vi "ECS-100X - Next Cycle Control.vi"(10 "CAS FPGA Ref":T1) -> ()   [LabVIEW 2015, in "ECS-RT.lvlib"]
uses:
  ECS-RT.lvlib
  <vilib>/addons/Combustion Analysis System/FPGA/CAS - FGPA - Reference.ctl
  Typedefs/MISC/50% MFB - Results.ctl
  <vilib>/addons/Combustion Analysis System/Real-Time/Globals/CAS - Control.vi
  Globals/RT Data.vi
  <vilib>/addons/Combustion Analysis System/Real-Time/Globals/Results/CAS - Results - All Results.vi
  <vilib>/addons/Combustion Analysis System/Real-Time/Globals/CAS - Queues.vi
  <vilib>/addons/Combustion Analysis System/Real-Time/Globals/Setup/CAS - Setup - Engine Geometry.vi
  Globals/Next Cycle Globals.vi
  <vilib>/Utility/error.llb/Error Cluster From Error Code.vi
  <vilib>/rvi/errors/niLvFpgaAdjustHostInterfaceError.vi
  <vilib>/rvi/interface/nirviReadWriteControl/nirviReadWriteControl.xnode
  ECS-Shared.lvlib
  NiFpgaLv.dll
  <vilib>/rvi/interface/Simulation/niFpgaSimulationCallBeginRW.vi
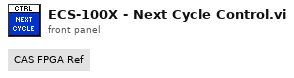
[diagram p1: front panel]
types:
  T1 = typedef "CAS - FGPA - Reference.ctl" = refnum<k20>
  T2 = typedef "ECS-Shared.lvlib/RT Data.ctl" = cluster{"Refs":T3, "EPT":T5, "Raw Inputs":T7, "Control Inputs":T14, "Control Outputs":T17, "Raw Outputs":T20}
  T3 = typedef "ECS-Shared.lvlib/FPGA Refs.ctl" = cluster{"FPGA 1":T4, "FPGA 2":T4}
  T4 = typedef "ECS-Shared.lvlib/Generic FPGA Ref.ctl" = refnum<k20>
  T5 = typedef "ECS-Shared.lvlib/EPT Cluster.ctl" = cluster{"MaxCAD":sgl, "EPT Sim Enabled":bool, "EPTxData":T6}
  T6 = typedef "EPTx - RevA - RT.lvlib/EPTxData.ctl" = cluster{"Sync":bool, "CurrentCAD":sgl, "Speed [RPM]":sgl, "Config":bool, "Rcvg Primary":bool, "Stall":bool, "Overflow":bool, "Ratio Error":bool, "Pattern Error":bool, "Aux Warning":bool, "Watchdog Error":bool}
  T7 = typedef "ECS-Shared.lvlib/Raw Inputs.ctl" = cluster{"NI9752s":T8[], "NI9757s":T10[], "NI9411s":T11[], "NI9220s":T12[], "VRHalls":T13[]}
  T8 = typedef "ECS-Shared.lvlib/NI9752.ctl" = cluster{"Voltage [V]":sgl[], "Resistance [Ohm]":sgl[], "PPWData VR1":T9, "PPWData VR2":T9, "PPWData Hall1":T9, "PPWData Hall2":T9}
  T9 = typedef "ECS-Shared.lvlib/PPWData.ctl" = cluster{"Period":u32, "PulseWidth":u32, "Stopped":bool}
  T10 = typedef "ECS-Shared.lvlib/NI9757.ctl" = cluster{"UEGO1":cluster{"Lambda":sgl, "Phi":sgl, "AF_Ratio":sgl, "Ip":sgl, "Temp":sgl, "Hot":bool}, "UEGO2":cluster{"Lambda":sgl, "Phi":sgl, "AF_Ratio":sgl, "Ip":sgl, "Temp":sgl, "Hot":bool}, "EGO1":cluster{"Status":enum16{"COLD SENSOR", "FOULED SENSOR", "RICH", "LEAN"}, "SensorV":sgl}, "EGO2":cluster{"Status":enum16{"COLD SENSOR", "FOULED SENSOR", "RICH", "LEAN"}, "SensorV":sgl}, "EGO3":cluster{"Status":enum16{"COLD SENSOR", "FOULED SENSOR", "RICH", "LEAN"}, "SensorV":sgl}, "EGO4":cluster{"Status":enum16{"COLD SENSOR", "FOULED SENSOR", "RICH", "LEAN"}, "SensorV":sgl}}
  T11 = typedef "ECS-Shared.lvlib/NI9411.ctl" = cluster{"PPWData 0":T9, "PPWData 1":T9, "PPWData 2":T9, "PPWData 3":T9, "PPWData 4":T9, "PPWData 5":T9}
  T12 = typedef "ECS-Shared.lvlib/NI9220.ctl" = cluster{"AI 0":sgl, "AI 1":sgl, "AI 2":sgl, "AI 3":sgl, "AI 4":sgl, "AI 5":sgl, "AI 6":sgl, "AI 7":sgl, "AI 8":sgl, "AI 9":sgl, "AI 10":sgl, "AI 11":sgl, "AI 12":sgl, "AI 13":sgl, "AI 14":sgl, "AI 15":sgl}
  T13 = typedef "ECS-Shared.lvlib/VRHall.ctl" = cluster{"PPWData 0":T9, "PPWData 1":T9, "PPWData 2":T9, "PPWData 3":T9, "PPWData 4":T9, "PPWData 5":T9}
  T14 = typedef "ECS-Shared.lvlib/Control Inputs.ctl" = cluster{"Engine Speed [RPM]":sgl, "Engine Status":T15, "Load Control \nMode":T16, "dt(s)":sgl, "Number of Cylinders":u8, "Engine Displacement [cc]":sgl, "StoichAFR":sgl, "Q.LHV Fuel [kJ/kg]":sgl, "BattV PSU [V]":sgl, "12V PSU [V]":sgl, "5V PSU [V]":sgl, "Pedal Position [%]":sgl, "Oil Pressure [kPa]":sgl, "Oil Temp [C]":sgl, "Oil Level [%]":sgl, "Engine Coolant Temp (ECT) [C]":sgl, "Engine Coolant Pressure [kPa]":sgl, "Rail Pressure [bar]":sgl, "Fuel Pressure [kPa]":sgl, "Fuel Temp [C]":sgl, "Vacuum Pressure [kPa]":sgl, "Throttle Position [%]":sgl, "Cam1 Advance [CAD]":sgl, "Cam2 Advance [CAD]":sgl, "Cam3 Advance [CAD]":sgl, "Cam4 Advance [CAD]":sgl, "CA50 Control Output [CAD]":sgl[], "CA50 Control Output Valid":bool[], "Intake Air Temp (IAT) [C]":sgl, "Barometric Air Pressure [kPa]":sgl, "Intake Air Rel. Humidity [%]":sgl, "Mass Air Flow (MAF) [kg/hr]":sgl, "Turbo Inlet Air Pressure [kPa]":sgl, "Turbo Inlet Air Temp [C]":sgl, "Turbo Outlet Air Pressure [kPa]":sgl, "Turbo Outlet Air Temp [C]":sgl, "CAC Outlet Pressure [kPa]":sgl, "CAC Outlet Temp [C]":sgl, "Intake Manifold Pressure (MAP) [kPa]":sgl, "Intake Manifold Temp (MAT) [C]":sgl, "Exhaust Manifold Pressure [kPa]":sgl, "Exhaust Manifold Temp [C]":sgl, "HighP EGR Cooler Outlet Pressure [kPa]":sgl, "HighP EGR Cooler Outlet Temp [C]":sgl, "HighP EGR Differential Pressure [kPa]":sgl, "HighP EGR Valve Position [%]":sgl, "Turbo Outlet Exhaust Pressure [kPa]":sgl, "Turbo Outlet Exhaust Temp [C]":sgl, "VGT Position 1 [%]":sgl, "VGT Position 2 [%]":sgl, "Turbo Speed 1 [RPM]":sgl, "Turbo Speed 2 [RPM]":sgl, "LowP EGR Differential Pressure [kPa]":sgl, "LowP EGR Valve Position [%]":sgl, "UEGO1Lambda":sgl, "UEGO1_Hot":bool, "UEGO2Lambda":sgl, "UEGO2_Hot":bool, "Knock Intensity":sgl[], "Knock":bool[]}
  T15 = typedef "ECS-Shared.lvlib/Engine Status.ctl" = enum16{"OFF", "STALLED", "CRANKING", "RUNNING", "ACCEL", "DECEL", "SAFE"}
  T16 = typedef "ECS-Shared.lvlib/Load Control Mode.ctl" = enum16{"No Governor", "Min Speed Governor", "Max Speed Governor"}
  T17 = typedef "ECS-Shared.lvlib/Control Outputs.ctl" = cluster{"Pedal Desired [%]":sgl, "MEP Desired [bar]":sgl, "Fuel Desired [mg/cyc]":sgl, "Intake MAP Desired [kPa]":sgl, "Cam1 Advance Setpoint [CAD]":sgl, "Cam2 Advance Setpoint [CAD]":sgl, "HighP EGR Position Setpoint [%Open]":sgl, "LowP EGR Position Setpoint [%Open]":sgl, "Rail Pressure Setpoint [bar]":sgl, "Wastegate1 Position Setpoint [%Open]":sgl, "Wastegate2 Position Setpoint [%Open]":sgl, "VGT1 Position Setpoint [%Open]":sgl, "VGT2 Position Setpoint [%Open]":sgl, "Throttle1 Position Setpoint [%Open]":sgl, "Throttle2 Position Setpoint [%Open]":sgl, "TurboBPV Position Setpoint [%Open]":sgl, "Spark Dwells [msec]":sgl[], "Spark Timings [DBTDC]":sgl[], "PFI Quantities [mg/inj]":sgl[], "PFI Timings [DBTDC]":sgl[], "DI Quantities [mg/inj]":T18[], "DI Timings [DBTDC]":T19[]}
  T18 = typedef "ECS-Shared.lvlib/Injection Quantity.ctl" = cluster{"Pilot1Quantity [mg/inj]":sgl, "Pilot2Quantity [mg/inj]":sgl, "MainQuantity [mg/inj]":sgl, "Post1Quantity [mg/inj]":sgl, "Post2Quantity [mg/inj]":sgl}
  T19 = typedef "ECS-Shared.lvlib/Injection Timing.ctl" = cluster{"Pilot1SOI [DBTDC]":sgl, "Pilot2SOI [DBTDC]":sgl, "MainSOI [DBTDC]":sgl, "Post1SOI [DBTDC]":sgl, "Post2SOI [DBTDC]":sgl}
  T20 = typedef "ECS-Shared.lvlib/Raw Outputs.ctl" = cluster{"9751-1":T21, "9751-2":T21, "9751-3":T21, "9751-4":T21, "9754-1":T23, "9754-2":T23, "9758-1":T25, "9758-2":T25, "9759-1":T28}
  T21 = typedef "ECS-Shared.lvlib/NI9751.ctl" = cluster{"DI1":T22, "DI2":T22, "DI3":T22}
  T22 = typedef "ECS-Shared.lvlib/DI.ctl" = cluster{"Window_Start (DBTDC)":sgl, "Window_End (DBTDC)":sgl, "Enable_Inj1":bool, "Duration_Inj1 (msec)":sgl, "Timing_Inj1 (DBTDC)":sgl, "Enable_Inj2":bool, "Duration_Inj2 (msec)":sgl, "Timing_Inj2 (DBTDC)":sgl, "Enable_Inj3":bool, "Duration_Inj3 (msec)":sgl, "Timing_Inj3 (DBTDC)":sgl, "Enable_Inj4":bool, "Duration_Inj4 (msec)":sgl, "Timing_Inj4 (DBTDC)":sgl, "Enable_Inj5":bool, "Duration_Inj5 (msec)":sgl, "Timing_Inj5 (DBTDC)":sgl}
  T23 = typedef "ECS-Shared.lvlib/NI9754.ctl" = cluster{"ESTTL 1":T24, "ESTTL 2":T24, "ESTTL 3":T24, "ESTTL 4":T24, "ESTTL 5":T24, "ESTTL 6":T24, "ESTTL 7":T24, "ESTTL 8":T24}
  T24 = typedef "ECS-Shared.lvlib/ESTTL.ctl" = cluster{"Timing (DBTDC)":sgl, "Dwell (ms)":sgl}
  T25 = typedef "ECS-Shared.lvlib/NI9758.ctl" = cluster{"LS 1":T26, "LS 2":T26, "LS 3":T26, "LS 4":T26, "PFI 1":T27, "PFI 2":T27, "PFI 3":T27, "PFI 4":T27}
  T26 = typedef "ECS-Shared.lvlib/LS.ctl" = cluster{"Enable":bool, "Freq [Hz]":sgl, "DutyCyc [%]":sgl}
  T27 = typedef "ECS-Shared.lvlib/PFI.ctl" = cluster{"Position Mode":bool, "Timing (DBTDC)":sgl, "Pulse Width (ms)":sgl}
  T28 = typedef "ECS-Shared.lvlib/NI9759.ctl" = cluster{"THR1-1 DC [%]":sgl, "THR1-1 Setpoint [% Open]":sgl, "THR1-2 DC [%]":sgl, "THR1-2 Setpoint [% Open]":sgl}
  T29 = cluster{"Start Time [ns]":u64, "FPGA Time [ns]":u64, "Cycle":u32, "Cycle Period [Ticks]":u32}
  T30 = typedef "ECS-Shared.lvlib/50% MFB - Results.ctl" = cluster{"Result Valid":bool, "Time [ns]":u64, "50% Mass Fraction [CAD]":sgl, "Current Angle [DBTDC]":sgl}
  T31 = typedef "CAS - Results - All Results.ctl" = cluster{"Cycle Results":T32, "Pegging Results":T33, "Basic Results":T34, "Mean Effective Pressure Results":T35, "Injection Results":T36, "Spark Results":T37, "Heat Release Results":T38, "Combustion Noise Results":T39, "Misfire Results":T40, "Cam Results":T41, "Synchronous Pump Results":T42, "PWM Results":T43[], "Knock Results":T44, "FPGA Results":T45[], "Medium Speed Results":T46[], "User Results":T47[], "Slow Speed Results":T48[]}
  T32 = typedef "CAS - Results - Cycle.ctl" = cluster{"Enabled":bool, "Error Code":i32, "Cylinder":i32, "Speed [RPM]":sgl, "Time [ns]":u64, "Cycle":u32}
  T33 = typedef "CAS - Results - Pegging.ctl" = cluster{"Enabled":bool, "Error Code":i32, "Pegging Value [kPa]":sgl}
  T34 = typedef "CAS - Results - Basic.ctl" = cluster{"Enabled":bool, "Error Code":i32, "Peak Pressure [kPa abs]":sgl[], "Peak Pressure Location [CAD]":sgl[], "Max Pressure Rise Rate [kPa/CAD]":sgl[], "Max Pressure Rise Rate Location [CAD]":sgl[], "Polytropic Compression":sgl[], "Polytropic Expansion":sgl[], "Intake Pressure [kPa abs]":sgl, "Exhaust Pressure [kPa abs]":sgl, "TDC Probe Location [CAD]":sgl}
  T35 = typedef "CAS - Results - Mean Effective Pressure.ctl" = cluster{"Enabled":bool, "Error Code":i32, "Gross Mean Effective Pressure [kPa]":sgl[], "Pumping Mean Effective Pressure [kPa]":sgl, "Net Mean Effective Pressure [kPa]":sgl, "Indicated Power [kW]":sgl}
  T36 = typedef "CAS - Results - Injection.ctl" = cluster{"Enabled":bool, "Error Code":i32, "Number of Injections":u8, "Start of Injection [CAD]":sgl[], "Injection Duration [ms]":sgl[], "Injection Fuel Flow [mg/Inj]":sgl[], "Cycle Fuel Flow [mg/Cycle]":sgl}
  T37 = typedef "CAS - Results - Spark.ctl" = cluster{"Enabled":bool, "Error Code":i32, "Number of Sparks":u8, "Spark [CAD]":sgl[], "Dwell [ms]":sgl[], "Restrikes":sgl[], "Restrike Delay [ms]":sgl[], "Restrike Dwell [ms]":sgl[]}
  T38 = typedef "CAS - Results - Heat Release.ctl" = cluster{"Enabled":bool, "Error Code":i32, "5% Mass Fraction Burned [CAD]":sgl[], "10% Mass Fraction Burned [CAD]":sgl[], "50% Mass Fraction Burned [CAD]":sgl[], "75% Mass Fraction Burned [CAD]":sgl[], "90% Mass Fraction Burned [CAD]":sgl[], "Max Heat Release Rate [J/CAD]":sgl[], "Max Heat Release Rate Location [CAD]":sgl[]}
  T39 = typedef "CAS - Results - Combustion Noise.ctl" = cluster{"Enabled":bool, "Error Code":i32, "Noise [db]":sgl}
  T40 = typedef "CAS - Results - Misfire.ctl" = cluster{"Enabled":bool, "Error Code":i32, "Misfire":sgl}
  T41 = typedef "CAS - Results - Cam.ctl" = cluster{"Enabled":bool, "Error Code":i32, "Intake Cam Phase [CAD]":sgl, "Intake Phase [CAD]":sgl[], "Exhaust Cam Phase [CAD]":sgl, "Exhaust Phase [CAD]":sgl[]}
  T42 = typedef "CAS - Results - Synchronous Pump.ctl" = cluster{"Enabled":bool, "Error Code":i32, "Number of Pumps":u8, "Pump Start [CAD]":sgl[], "Pump End [CAD]":sgl[], "Pump Duration [CAD]":sgl[]}
  T43 = typedef "CAS - Results - PWM.ctl" = cluster{"Name":string, "Value":sgl}
  T44 = typedef "CAS - Results - Knock.ctl" = cluster{"Enabled":bool, "Error Code":i32, "Knock":sgl, "Peak-To-Peak":sgl}
  T45 = typedef "CAS - Results - FPGA.ctl" = cluster{"Name":string, "Value":sgl}
  T46 = typedef "CAS - Results - Medium Speed.ctl" = cluster{"Name":string, "Value":sgl}
  T47 = typedef "CAS - Results - User.ctl" = cluster{"Name":string, "Value":sgl}
  T48 = typedef "CAS - Results - Slow Speed.ctl" = cluster{"Name":string, "Value":sgl}
  T49 = typedef "DCAT.lvlib/DCAT - Results - All Results.ctl" = cluster{"Cycle Results":T50, "Pegging Results":T51, "Basic Results":T52, "Mean Effective Pressure Results":T53, "Injection Results":T54, "Spark Results":T55, "Heat Release Results":T56, "Combustion Noise Results":T57, "Misfire Results":T58, "Cam Results":T59, "Synchronous Pump Results":T60, "PWM Results":T61[], "Knock Results":T62, "FPGA Results":T63[], "Medium Speed Results":T64[], "User Results":T65[], "Slow Speed Results":T66[]}
  T50 = typedef "DCAT.lvlib/DCAT - Results - Cycle.ctl" = cluster{"Enabled":bool, "Error Code":i32, "Cylinder":i32, "Speed [RPM]":sgl, "Time [ns]":u64, "Cycle":u32}
  T51 = typedef "DCAT.lvlib/DCAT - Results - Pegging.ctl" = cluster{"Enabled":bool, "Error Code":i32, "Pegging Value [kPa]":sgl}
  T52 = typedef "DCAT.lvlib/DCAT - Results - Basic.ctl" = cluster{"Enabled":bool, "Error Code":i32, "Peak Pressure [kPa abs]":sgl[], "Peak Pressure Location [CAD]":sgl[], "Max Pressure Rise Rate [kPa/CAD]":sgl[], "Max Pressure Rise Rate Location [CAD]":sgl[], "Polytropic Compression":sgl[], "Polytropic Expansion":sgl[], "Intake Pressure [kPa abs]":sgl, "Exhaust Pressure [kPa abs]":sgl, "TDC Probe Location [CAD]":sgl}
  T53 = typedef "DCAT.lvlib/DCAT - Results - Mean Effective Pressure.ctl" = cluster{"Enabled":bool, "Error Code":i32, "Gross Mean Effective Pressure [kPa]":sgl[], "Pumping Mean Effective Pressure [kPa]":sgl, "Net Mean Effective Pressure [kPa]":sgl, "Indicated Power [kW]":sgl}
  T54 = typedef "DCAT.lvlib/DCAT - Results - Injection.ctl" = cluster{"Enabled":bool, "Error Code":i32, "Number of Injections":u8, "Start of Injection [CAD]":sgl[], "Injection Duration [ms]":sgl[], "Injection Fuel Flow [mg/Inj]":sgl[], "Cycle Fuel Flow [mg/Cycle]":sgl}
  T55 = typedef "DCAT.lvlib/DCAT - Results - Spark.ctl" = cluster{"Enabled":bool, "Error Code":i32, "Number of Sparks":u8, "Spark [CAD]":sgl[], "Dwell [ms]":sgl[], "Restrikes":sgl[], "Restrike Delay [ms]":sgl[], "Restrike Dwell [ms]":sgl[]}
  T56 = typedef "DCAT.lvlib/DCAT - Results - Heat Release.ctl" = cluster{"Enabled":bool, "Error Code":i32, "5% Mass Fraction Burned [CAD]":sgl[], "10% Mass Fraction Burned [CAD]":sgl[], "50% Mass Fraction Burned [CAD]":sgl[], "75% Mass Fraction Burned [CAD]":sgl[], "90% Mass Fraction Burned [CAD]":sgl[], "Max Heat Release Rate [J/CAD]":sgl[], "Max Heat Release Rate Location [CAD]":sgl[]}
  T57 = typedef "DCAT.lvlib/DCAT - Results - Combustion Noise.ctl" = cluster{"Enabled":bool, "Error Code":i32, "Noise [db]":sgl}
  T58 = typedef "DCAT.lvlib/DCAT - Results - Misfire.ctl" = cluster{"Enabled":bool, "Error Code":i32, "Misfire":sgl}
  T59 = typedef "DCAT.lvlib/DCAT - Results - Cam.ctl" = cluster{"Enabled":bool, "Error Code":i32, "Intake Cam Phase [CAD]":sgl, "Intake Phase [CAD]":sgl[], "Exhaust Cam Phase [CAD]":sgl, "Exhaust Phase [CAD]":sgl[]}
  T60 = typedef "DCAT.lvlib/DCAT - Results - Synchronous Pump.ctl" = cluster{"Enabled":bool, "Error Code":i32, "Number of Pumps":u8, "Pump Start [CAD]":sgl[], "Pump End [CAD]":sgl[], "Pump Duration [CAD]":sgl[]}
  T61 = typedef "DCAT.lvlib/DCAT - Results - PWM.ctl" = cluster{"Name":string, "Value":sgl}
  T62 = typedef "DCAT.lvlib/DCAT - Results - Knock.ctl" = cluster{"Enabled":bool, "Error Code":i32, "Knock":sgl, "Peak-To-Peak":sgl}
  T63 = typedef "DCAT.lvlib/DCAT - Results - FPGA.ctl" = cluster{"Name":string, "Value":sgl}
  T64 = typedef "DCAT.lvlib/DCAT - Results - Medium Speed.ctl" = cluster{"Name":string, "Value":sgl}
  T65 = typedef "DCAT.lvlib/DCAT - Results - User.ctl" = cluster{"Name":string, "Value":sgl}
  T66 = typedef "DCAT.lvlib/DCAT - Results - Slow Speed.ctl" = cluster{"Name":string, "Value":sgl}
  T67 = typedef "CAS - Setup - Engine Geometry.ctl" = cluster{"Engine":string, "Project":string, "Operator":string, "Rotations Per Cycle":u8, "Intake Valve Open [DATDC]":sgl, "Intake Valve Close [DATDC]":sgl, "Exhaust Valve Open [DATDC]":sgl, "Exhaust Valve Close [DATDC]":sgl, "Bore [m]":sgl, "Stroke [m]":sgl, "Connecting Rod Length [m]":sgl, "Pin Offset [m]":sgl, "Clearance Volume [liter]":sgl, "Max Speed [RPM]":sgl, "Head Area [%]":sgl, "Crown Area [%]":sgl, "Cylinder Count":u32, "Polytropic Exponent":sgl, "Polytropic Exponent Source":enum32{"Constant Value", "Calculated Value"}, "Volume File Enable":bool, "Volume File Path":path, "Cylinder TDC [DATDC]":sgl[], "Encoder Resolution [ppr]":u32, "Random Z":u8, "Digital Filter [us]":sgl, "Encoder Extrap Level":u8, "Encoder Divide":u32, "TDC Offset [CAD]":sgl, "Phase":enum32{"1 Z/Cycle", "Gate Z", "Random Z", "Reset Z"}, "Encoder Setup":enum32{"A Rising Edge", "A Any Edge", "A & B Any Edge"}, "Max Sync Rate [kS/s]":sgl, "Async Rate [kS/s]":sgl, "Medium Speed Rate [S/s]":sgl, "No FPGA":bool, "cDAQ DIO Module":tag, "Dynamic Start-Start":bool, "Start-Stop Rate [kS/s]":sgl}
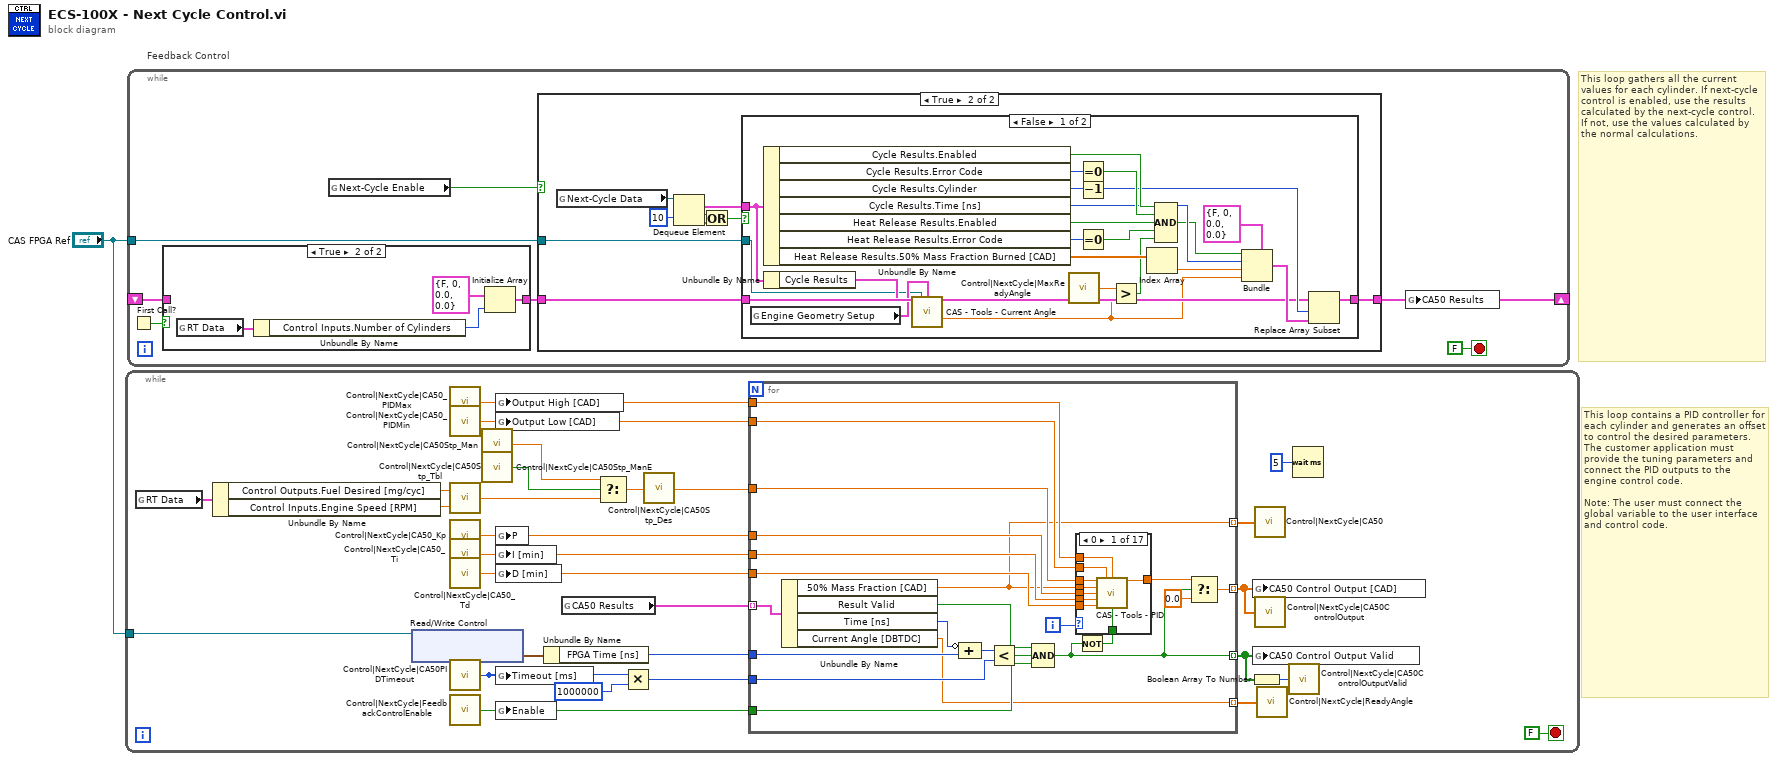
[diagram p0: block diagram]
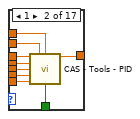
[diagram p2: hidden frame]
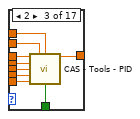
[diagram p3: hidden frame]
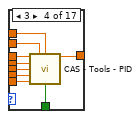
[diagram p4: hidden frame]
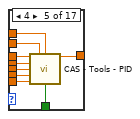
[diagram p5: hidden frame]
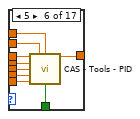
[diagram p6: hidden frame]
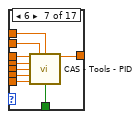
[diagram p7: hidden frame]
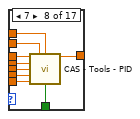
[diagram p8: hidden frame]
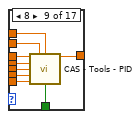
[diagram p9: hidden frame]
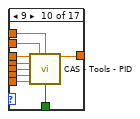
[diagram p10: hidden frame]
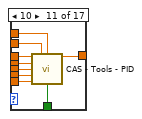
[diagram p11: hidden frame]
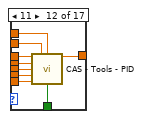
[diagram p12: hidden frame]
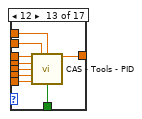
[diagram p13: hidden frame]
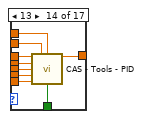
[diagram p14: hidden frame]
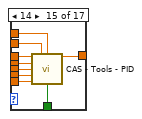
[diagram p15: hidden frame]
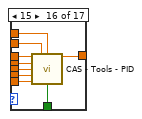
[diagram p16: hidden frame]
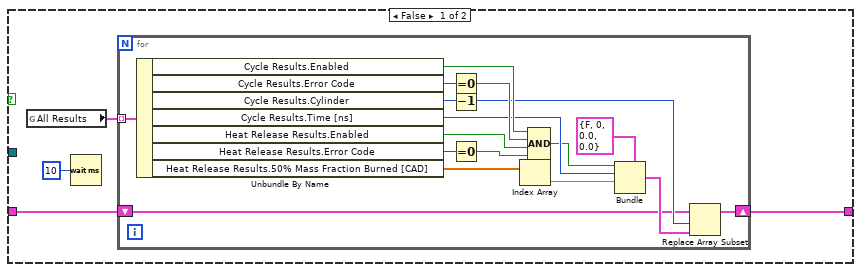
[diagram p19: hidden frame]
diagram:
  # "This loop contains a PID controller for each cylinder and generates an offset to control the desired parameters. The customer application must provide the tuning parameters and connect the PID outputs to the engine control code.\n\nNote: The user must connect the global variable to the user interface and control code."
  # "This loop gathers all the current values for each cylinder. If next-cycle control is enabled, use the results calculated by the next-cycle control. If not, use the values calculated by the normal calculations."
  # "Feedback Control"
  n1 = while {
    tunnel: "CAS FPGA Ref" -> [w25]
    stop <- FALSE stop-if-true
    n2 = global read "RT Data.vi" "RT Data"() -> (w4:T2)
    n3 = Unbundle By Name(w4) -> ("Control Outputs.Fuel Desired [mg/cyc]"=w2:sgl, "Control Inputs.Engine Speed [RPM]"=w3:sgl)
    n4 = xnode "Read/Write Control"("FPGA VI Reference In"=w25) -> ("CAS-Sample Data"=w24:T29)  [unwired: 1 in, 2 out]
    n5 = call "Control|NextCycle|CA50_PIDMax"() -> ("Value"=w17:sgl)
    n6 = call "Control|NextCycle|CA50_PIDMin"() -> ("Value"=w16:sgl)
    n7 = call "Control|NextCycle|CA50Stp_Tbl"("Y Index"=w3, "X Index"=w2) -> ("Z"=w11:sgl)
    n8 = call "Control|NextCycle|CA50_Kp"() -> ("Value"=w20:sgl)
    n9 = call "Control|NextCycle|CA50_Ti"() -> ("Value"=w19:sgl)
    n10 = call "Control|NextCycle|CA50_Td"() -> ("Value"=w18:sgl)
    n11 = call "Control|NextCycle|CA50PIDTimeout"() -> ("Value"=w15:u32)
    n12 = call "Control|NextCycle|FeedbackControlEnable"() -> ("Value"=w14:bool)
    n13 = call "Control|NextCycle|CA50Stp_Man"() -> ("Value"=w13:sgl)
    n14 = call "Control|NextCycle|CA50Stp_ManE"() -> ("Value"=w12:bool)
    n15 = global write "Next Cycle Globals.vi" "Output High [CAD]"(w17) -> ()
    n16 = global write "Next Cycle Globals.vi" "Output Low [CAD]"(w16) -> ()
    n17 = global write "Next Cycle Globals.vi" "P"(w20) -> ()
    n18 = global write "Next Cycle Globals.vi" "I [min]"(w19) -> ()
    n19 = global write "Next Cycle Globals.vi" "D [min]"(w18) -> ()
    n20 = global write "Next Cycle Globals.vi" "Timeout [ms]"(w15) -> ()
    n21 = global write "Next Cycle Globals.vi" "Enable"(w14) -> ()
    n22 = Unbundle By Name(w24) -> ("FPGA Time [ns]"=w23:u64)
    n23 = global read "Next Cycle Globals.vi" "CA50 Results"() -> (w26:T30[])
    n24 = Select(t=w13, s=w12, f=w11) -> (s? t:f=w10:sgl)
    n25 = Multiply(x=w15, y=u32 1000000) -> (x*y=w22:u32)
    n26 = call "Control|NextCycle|CA50Stp_Des"("Value"=w10) -> ()
    n27 = for {
      tunnel: w26 -> [w47] mode=indexing
      tunnel: [w48] -> w7 mode=indexing
      tunnel: w23 -> [w45]
      tunnel: w22 -> [w42]
      tunnel: w17 -> [w40]
      tunnel: w16 -> [w39]
      tunnel: w10 -> [w38]
      tunnel: w20 -> [w37]
      tunnel: w19 -> [w36]
      tunnel: w18 -> [w35]
      tunnel: [w32] -> w9 mode=indexing
      tunnel: w14 -> [w31]
      tunnel: [w30] -> w6 mode=indexing
      tunnel: [w29] -> w5 mode=indexing
      i -> [w41]
      n28 = Unbundle By Name(w47) -> ("50% Mass Fraction [CAD]"=w30:sgl, "Result Valid"=w33:bool, "Time [ns]"=w46:u64, "Current Angle [DBTDC]"=w29:sgl)
      n29 = Compound Arithmetic op=ADD(invert w46, w45) -> (w44:u64)
      n30 = Less?(x=w44, y=w42) -> (x < y?=w43:bool)
      n31 = Compound Arithmetic op=AND(w33, w43, w31) -> (w32:bool)
      n32 = Not(x=w32) -> (.not. x?=w34:bool)
      n33 = case shown="0" w41 {
        tunnel: w34 -> [w56 w65 w74 w83 w92 w101 w110 w119 w128 w137 w146 w155 w164 w173 w182 w191 _]
        tunnel: [w58 w67 w76 w85 w94 w103 w112 w121 w130 w139 w148 w157 w166 w175 w184 w193 _] -> w50
        tunnel: w30 -> [w59 w68 w77 w86 w95 w104 w113 w122 w131 w140 w149 w158 w167 w176 w185 w194 _]
        tunnel: w38 -> [w57 w66 w75 w84 w93 w102 w111 w120 w129 w138 w147 w156 w165 w174 w183 w192 _]
        tunnel: w37 -> [w55 w64 w73 w82 w91 w100 w109 w118 w127 w136 w145 w154 w163 w172 w181 w190 _]
        tunnel: w36 -> [w54 w63 w72 w81 w90 w99 w108 w117 w126 w135 w144 w153 w162 w171 w180 w189 _]
        tunnel: w35 -> [w53 w62 w71 w80 w89 w98 w107 w116 w125 w134 w143 w152 w161 w170 w179 w188 _]
        tunnel: w39 -> [w52 w61 w70 w79 w88 w97 w106 w115 w124 w133 w142 w151 w160 w169 w178 w187 _]
        tunnel: w40 -> [w51 w60 w69 w78 w87 w96 w105 w114 w123 w132 w141 w150 w159 w168 w177 w186 _]
        frame 0 {
          n34 = call <vilib>:"CAS - Tools - PID.vi"("Setpoint"=w57, "OutputLow"=w52, "OutputHigh"=w51, "ProcessVariable"=w59, "ProportionalGain (Kc)"=w55, "IntegralTime (Ti, min)"=w54, "DerivativeTime (Td, min)"=w53, "Reinitialize? (F)"=w56) -> ("Output"=w58:sgl)  [unwired: 2 in, 5 out]
        }
        frame 1 {
          n35 = call <vilib>:"CAS - Tools - PID.vi"("Setpoint"=w66, "OutputLow"=w61, "OutputHigh"=w60, "ProcessVariable"=w68, "ProportionalGain (Kc)"=w64, "IntegralTime (Ti, min)"=w63, "DerivativeTime (Td, min)"=w62, "Reinitialize? (F)"=w65) -> ("Output"=w67:sgl)  [unwired: 2 in, 5 out]
        }
        frame 2 {
          n36 = call <vilib>:"CAS - Tools - PID.vi"("Setpoint"=w75, "OutputLow"=w70, "OutputHigh"=w69, "ProcessVariable"=w77, "ProportionalGain (Kc)"=w73, "IntegralTime (Ti, min)"=w72, "DerivativeTime (Td, min)"=w71, "Reinitialize? (F)"=w74) -> ("Output"=w76:sgl)  [unwired: 2 in, 5 out]
        }
        frame 3 {
          n37 = call <vilib>:"CAS - Tools - PID.vi"("Setpoint"=w84, "OutputLow"=w79, "OutputHigh"=w78, "ProcessVariable"=w86, "ProportionalGain (Kc)"=w82, "IntegralTime (Ti, min)"=w81, "DerivativeTime (Td, min)"=w80, "Reinitialize? (F)"=w83) -> ("Output"=w85:sgl)  [unwired: 2 in, 5 out]
        }
        frame 4 {
          n38 = call <vilib>:"CAS - Tools - PID.vi"("Setpoint"=w93, "OutputLow"=w88, "OutputHigh"=w87, "ProcessVariable"=w95, "ProportionalGain (Kc)"=w91, "IntegralTime (Ti, min)"=w90, "DerivativeTime (Td, min)"=w89, "Reinitialize? (F)"=w92) -> ("Output"=w94:sgl)  [unwired: 2 in, 5 out]
        }
        frame 5 {
          n39 = call <vilib>:"CAS - Tools - PID.vi"("Setpoint"=w102, "OutputLow"=w97, "OutputHigh"=w96, "ProcessVariable"=w104, "ProportionalGain (Kc)"=w100, "IntegralTime (Ti, min)"=w99, "DerivativeTime (Td, min)"=w98, "Reinitialize? (F)"=w101) -> ("Output"=w103:sgl)  [unwired: 2 in, 5 out]
        }
        frame 6 {
          n40 = call <vilib>:"CAS - Tools - PID.vi"("Setpoint"=w111, "OutputLow"=w106, "OutputHigh"=w105, "ProcessVariable"=w113, "ProportionalGain (Kc)"=w109, "IntegralTime (Ti, min)"=w108, "DerivativeTime (Td, min)"=w107, "Reinitialize? (F)"=w110) -> ("Output"=w112:sgl)  [unwired: 2 in, 5 out]
        }
        frame 7 {
          n41 = call <vilib>:"CAS - Tools - PID.vi"("Setpoint"=w120, "OutputLow"=w115, "OutputHigh"=w114, "ProcessVariable"=w122, "ProportionalGain (Kc)"=w118, "IntegralTime (Ti, min)"=w117, "DerivativeTime (Td, min)"=w116, "Reinitialize? (F)"=w119) -> ("Output"=w121:sgl)  [unwired: 2 in, 5 out]
        }
        frame 8 {
          n42 = call <vilib>:"CAS - Tools - PID.vi"("Setpoint"=w129, "OutputLow"=w124, "OutputHigh"=w123, "ProcessVariable"=w131, "ProportionalGain (Kc)"=w127, "IntegralTime (Ti, min)"=w126, "DerivativeTime (Td, min)"=w125, "Reinitialize? (F)"=w128) -> ("Output"=w130:sgl)  [unwired: 2 in, 5 out]
        }
        frame 9 {
          n43 = call <vilib>:"CAS - Tools - PID.vi"("Setpoint"=w138, "OutputLow"=w133, "OutputHigh"=w132, "ProcessVariable"=w140, "ProportionalGain (Kc)"=w136, "IntegralTime (Ti, min)"=w135, "DerivativeTime (Td, min)"=w134, "Reinitialize? (F)"=w137) -> ("Output"=w139:sgl)  [unwired: 2 in, 5 out]
        }
        frame 10 {
          n44 = call <vilib>:"CAS - Tools - PID.vi"("Setpoint"=w147, "OutputLow"=w142, "OutputHigh"=w141, "ProcessVariable"=w149, "ProportionalGain (Kc)"=w145, "IntegralTime (Ti, min)"=w144, "DerivativeTime (Td, min)"=w143, "Reinitialize? (F)"=w146) -> ("Output"=w148:sgl)  [unwired: 2 in, 5 out]
        }
        frame 11 {
          n45 = call <vilib>:"CAS - Tools - PID.vi"("Setpoint"=w156, "OutputLow"=w151, "OutputHigh"=w150, "ProcessVariable"=w158, "ProportionalGain (Kc)"=w154, "IntegralTime (Ti, min)"=w153, "DerivativeTime (Td, min)"=w152, "Reinitialize? (F)"=w155) -> ("Output"=w157:sgl)  [unwired: 2 in, 5 out]
        }
        frame 12 {
          n46 = call <vilib>:"CAS - Tools - PID.vi"("Setpoint"=w165, "OutputLow"=w160, "OutputHigh"=w159, "ProcessVariable"=w167, "ProportionalGain (Kc)"=w163, "IntegralTime (Ti, min)"=w162, "DerivativeTime (Td, min)"=w161, "Reinitialize? (F)"=w164) -> ("Output"=w166:sgl)  [unwired: 2 in, 5 out]
        }
        frame 13 {
          n47 = call <vilib>:"CAS - Tools - PID.vi"("Setpoint"=w174, "OutputLow"=w169, "OutputHigh"=w168, "ProcessVariable"=w176, "ProportionalGain (Kc)"=w172, "IntegralTime (Ti, min)"=w171, "DerivativeTime (Td, min)"=w170, "Reinitialize? (F)"=w173) -> ("Output"=w175:sgl)  [unwired: 2 in, 5 out]
        }
        frame 14 {
          n48 = call <vilib>:"CAS - Tools - PID.vi"("Setpoint"=w183, "OutputLow"=w178, "OutputHigh"=w177, "ProcessVariable"=w185, "ProportionalGain (Kc)"=w181, "IntegralTime (Ti, min)"=w180, "DerivativeTime (Td, min)"=w179, "Reinitialize? (F)"=w182) -> ("Output"=w184:sgl)  [unwired: 2 in, 5 out]
        }
        frame 15 {
          n49 = call <vilib>:"CAS - Tools - PID.vi"("Setpoint"=w192, "OutputLow"=w187, "OutputHigh"=w186, "ProcessVariable"=w194, "ProportionalGain (Kc)"=w190, "IntegralTime (Ti, min)"=w189, "DerivativeTime (Td, min)"=w188, "Reinitialize? (F)"=w191) -> ("Output"=w193:sgl)  [unwired: 2 in, 5 out]
        }
        frame Default {
        }
      }
      n50 = Select(t=w50, s=w32, f=sgl 0.0) -> (s? t:f=w48:sgl)
    }
    n51 = Boolean Array To Number(Boolean array=w9) -> (number=w8:u8)
    n52 = global write "Next Cycle Globals.vi" "CA50 Control Output [CAD]"(w7) -> ()
    n53 = global write "Next Cycle Globals.vi" "CA50 Control Output Valid"(w9) -> ()
    n54 = call "Control|NextCycle|CA50"("Value"=w6) -> ()
    n55 = call "Control|NextCycle|CA50ControlOutput"("Value"=w7) -> ()
    n56 = call "Control|NextCycle|ReadyAngle"("Value"=w5) -> ()
    n57 = call "Control|NextCycle|CA50ControlOutputValid"("Value"=w8) -> ()
    n58 = Wait (ms)(milliseconds to wait=u32 5) -> ()  [unwired: 1 out]
  }
  n59 = while {
    shift-right: [w199] -> _
    shift-left: _ -> [w197]
    tunnel: "CAS FPGA Ref" -> [w195]
    stop <- FALSE stop-if-true
    n60 = First Call?() -> (First Call?: T/F=w198:bool)
    n61 = case shown="True" w198 {
      tunnel: w197 -> [w202 _]
      tunnel: [w202 w205] -> w196
      frame False {
      }
      frame True {
        n62 = global read "RT Data.vi" "RT Data"() -> (w204:T2)
        n63 = Unbundle By Name(w204) -> ("Control Inputs.Number of Cylinders"=w203:u8)
        n64 = Initialize Array(T30 {"Result Valid"=FALSE, "Time [ns]"=0, "50% Mass Fraction [CAD]"=0.0, "Current Angle [DBTDC]"=0.0}, w203) -> (w205:T30[])
      }
    }
    n65 = global read "CAS - Control.vi" "Next-Cycle Enable"() -> (w200:bool)
    n66 = case shown="True" w200 {
      tunnel: w196 -> [w209 w229]
      tunnel: [w208 w230] -> w199
      tunnel: w195 -> [_ w228]
      frame False {
        n67 = global read "CAS - Results - All Results.vi" "All Results"() -> (w210:T31[])
        n68 = Wait (ms)(milliseconds to wait=u32 10) -> ()  [unwired: 1 out]
        n69 = for {
          tunnel: w210 -> [w211] mode=indexing
          shift-right: [w212] -> w208
          shift-left: w209 -> [w213]
          n70 = Unbundle By Name(w211) -> ("Cycle Results.Enabled"=w227:bool, "Cycle Results.Error Code"=w225:i32, "Cycle Results.Cylinder"=w220:i32, "Cycle Results.Time [ns]"=w216:u64, "Heat Release Results.Enabled"=w226:bool, "Heat Release Results.Error Code"=w223:i32, "Heat Release Results.50% Mass Fraction Burned [CAD]"=w221:sgl[])
          n71 = Equal To 0?(x=w225) -> (x = 0?=w224:bool)
          n72 = Decrement(x=w220) -> (x-1=w219:i32)
          n73 = Equal To 0?(x=w223) -> (x = 0?=w222:bool)
          n74 = Index Array(array=w221) -> (element=w215:sgl)  [unwired: 1 in]
          n75 = Compound Arithmetic op=AND(w227, w224, w226, w222) -> (w214:bool)
          n76 = Bundle(cluster=T30 {"Result Valid"=FALSE, "Time [ns]"=0, "50% Mass Fraction [CAD]"=0.0, "Current Angle [DBTDC]"=0.0}, "Result Valid"=w214, "Time [ns]"=w216, "50% Mass Fraction [CAD]"=w215) -> (w217:T30)  [unwired: 1 in]
          n77 = Replace Array Subset(array=w213, new element=w217, index=w219) -> (w212:T30[])
        }
      }
      frame True {
        n78 = global read "CAS - Queues.vi" "Next-Cycle Data"() -> (w236:refnum<queue>)
        n79 = Dequeue Element(queue=w236, timeout in ms (-1)=10) -> (element=w234:T49, timed out?=w233:bool, error out=w232:errorcluster)  [unwired: 1 in, 1 out]
        n80 = Or(x=w233, y=w232) -> (x .or. y?=w231:bool)
        n81 = case shown="False" w231 {
          tunnel: w234 -> [w243 _]
          tunnel: [w250 w260] -> w230
          tunnel: w229 -> [w245 w260]
          tunnel: w228 -> [w237 _]
          frame False {
            n82 = global read "CAS - Setup - Engine Geometry.vi" "Engine Geometry Setup"() -> (w241:T67)
            n83 = Unbundle By Name(w243) -> ("Cycle Results.Enabled"=w259:bool, "Cycle Results.Error Code"=w257:i32, "Cycle Results.Cylinder"=w252:i32, "Cycle Results.Time [ns]"=w247:u64, "Heat Release Results.Enabled"=w258:bool, "Heat Release Results.Error Code"=w255:i32, "Heat Release Results.50% Mass Fraction Burned [CAD]"=w253:sgl[])
            n84 = Unbundle By Name(w243) -> ("Cycle Results"=w242:T50)
            n85 = call <vilib>:"CAS - Tools - Current Angle.vi"("Cycle Results"=w242, "FPGA"=w237, "Engine Geometry Setup"=w241) -> ("Current Angle [CAD]"=w239:sgl)  [unwired: 11 in, 1 out]
            n86 = call "Control|NextCycle|MaxReadyAngle"() -> ("Value"=w240:sgl)
            n87 = Equal To 0?(x=w257) -> (x = 0?=w256:bool)
            n88 = Decrement(x=w252) -> (x-1=w251:i32)
            n89 = Equal To 0?(x=w255) -> (x = 0?=w254:bool)
            n90 = Greater?(x=w240, y=w239) -> (0:w238:bool)
            n91 = Index Array(array=w253) -> (element=w246:sgl)  [unwired: 1 in]
            n92 = Compound Arithmetic op=AND(w259, w256, w258, w254, w238) -> (w244:bool)
            n93 = Bundle(cluster=T30 {"Result Valid"=FALSE, "Time [ns]"=0, "50% Mass Fraction [CAD]"=0.0, "Current Angle [DBTDC]"=0.0}, "Result Valid"=w244, "Time [ns]"=w247, "50% Mass Fraction [CAD]"=w246, "Current Angle [DBTDC]"=w239) -> (w248:T30)
            n94 = Replace Array Subset(array=w245, new element=w248, index=w251) -> (w250:T30[])
          }
          frame True {
          }
        }
      }
    }
    n95 = global write "Next Cycle Globals.vi" "CA50 Results"(w199) -> ()
  }
